vi "OpenVIs.vi"(8 "error in (no error)":errorcluster, 9 "Title Prefix In":string, 10 "VI Screenshots":T1, 11 "VI Path":path) -> (0 "error out":errorcluster, 2 "VI Screenshots out":T1)   [LabVIEW 2020, in "VIDiffUtilities.lvlib"]
uses:
  VIDiffUtilities.lvlib
  Screenshots/VIScreenshots.ctl
  Screenshots/ScreenshotInfo.ctl
  Screenshots/Screenshot Type.ctl
  FilePaths.ctl
  Screenshots/VIDiffScreenshots.lvlib
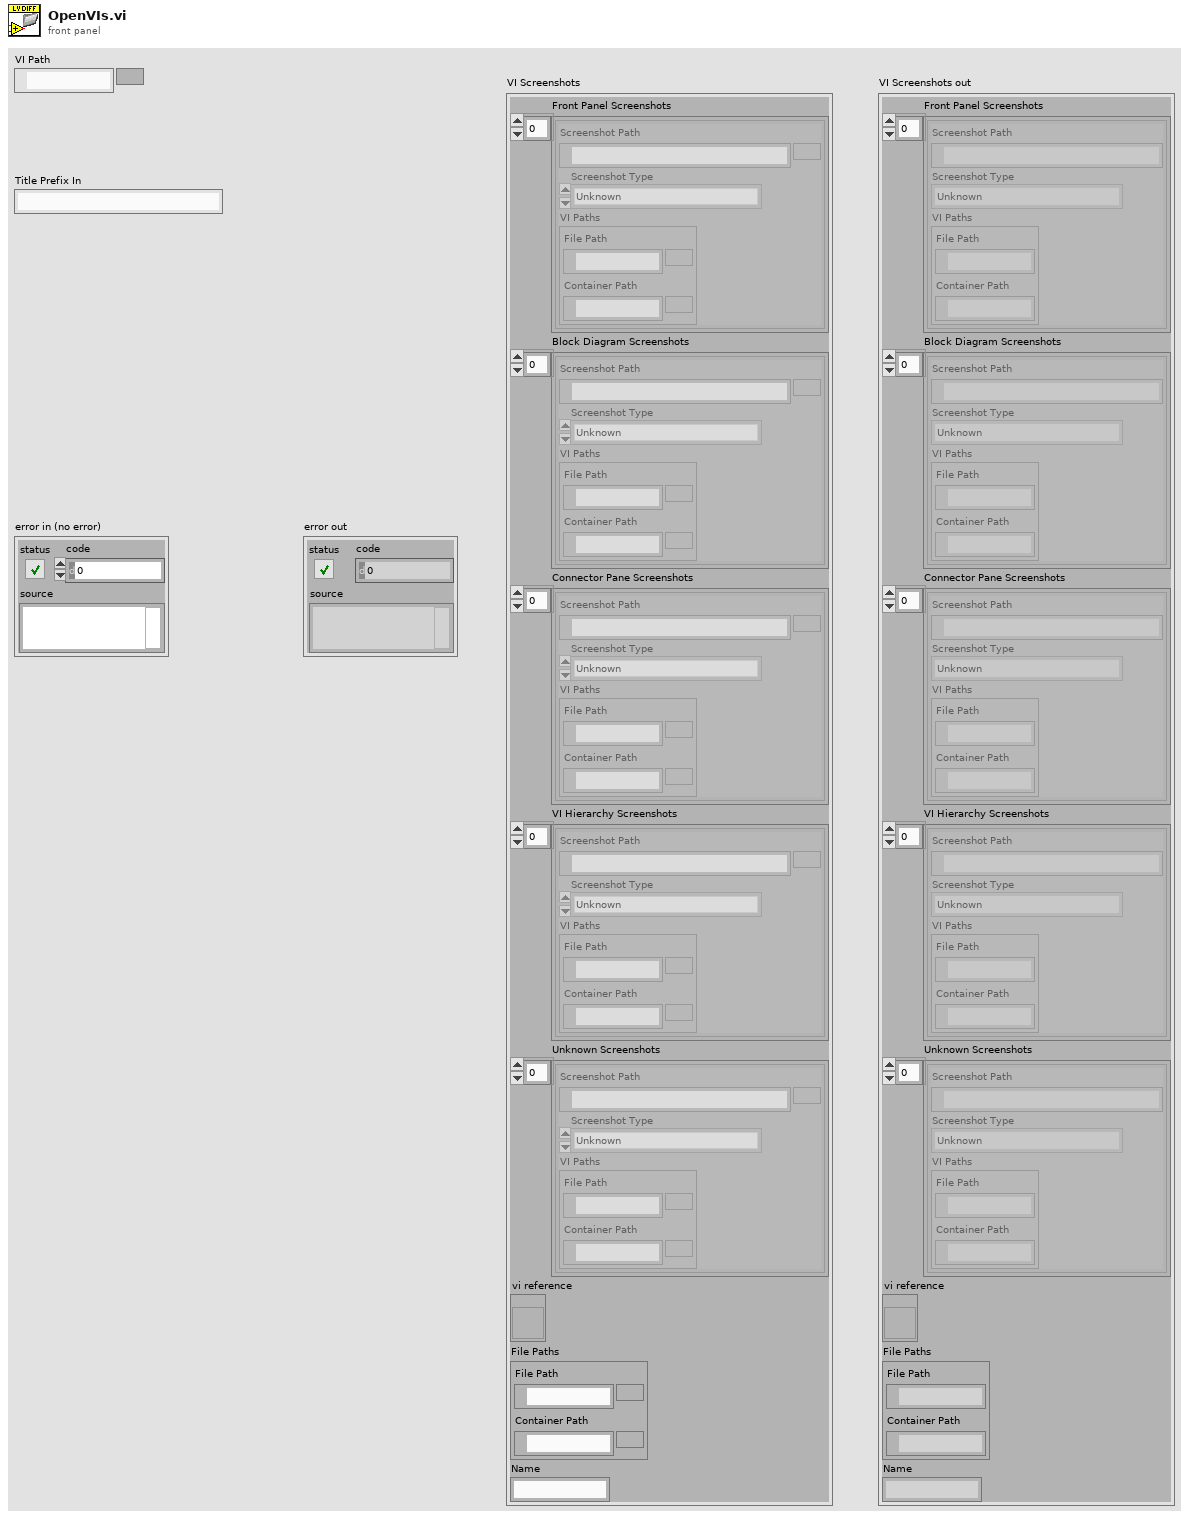
[diagram p1: front panel]
types:
  T1 = typedef "VIDiffScreenshots.lvlib/VIScreenshots.ctl" = cluster{"Front Panel Screenshots":T2[], "Block Diagram Screenshots":T2[], "Connector Pane Screenshots":T2[], "VI Hierarchy Screenshots":T2[], "Unknown Screenshots":T2[], "vi reference":refnum<vi>, "File Paths":cluster{"File Path":path, "Container Path":path}, "Name":string}
  T2 = typedef "VIDiffScreenshots.lvlib/ScreenshotInfo.ctl" = cluster{"Screenshot Path":path, "Screenshot Type":T3, "VI Paths":T4}
  T3 = typedef "VIDiffScreenshots.lvlib/Screenshot Type.ctl" = enum16{"Unknown", "Front Panel", "Connector Pane", "Block Diagram", "VI Hierarchy"}
  T4 = typedef "VIDiffUtilities.lvlib/FilePaths.ctl" = cluster{"File Path":path, "Container Path":path}
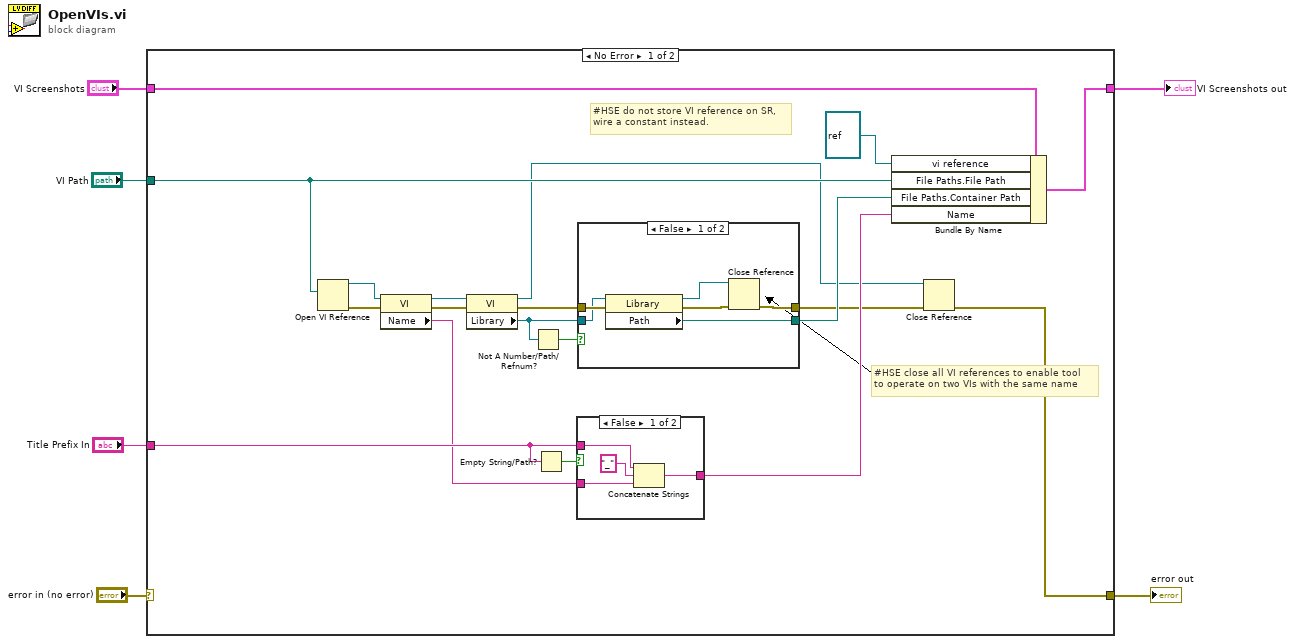
[diagram p0: block diagram]
diagram:
  n1 = case shown="No Error" "error in (no error)" {
    selector: "error in (no error)" -> [_ w39]
    tunnel: [w8 w39] -> w5
    tunnel: "VI Screenshots" -> [w22 w38]
    tunnel: [w20 w38] -> w3
    tunnel: "VI Path" -> [w19 _]
    tunnel: "Title Prefix In" -> [w13 _]
    frame No Error {
      # "#HSE do not store VI reference on SR,\nwire a constant instead."
      # "#HSE close all VI references to enable tool \nto operate on two VIs with the same name"
      n2 = Open VI Reference(vi path=w19) -> (vi reference=w18:refnum<vi>, error out=w17:errorcluster)  [unwired: 5 in]
      n3 = property class="VI"(reference=w18, error in=w17) -> (reference out=w15:refnum<vi>, error out=w16:errorcluster, "Name"=w12:string)
      n4 = property class="VI"(reference=w15, error in=w16) -> (reference out=w10:refnum<vi>, error out=w25:errorcluster, "Library"=w23:refnum<vi>)
      n5 = Not A Number/Path/Refnum?(number/path/refnum=w23) -> (NaN/Path/Refnum?=w24:bool)
      n6 = Empty String/Path?(string/path=w13) -> (empty?=w14:bool)
      n7 = case shown="False" w14 {
        tunnel: w12 -> [w29 w30]
        tunnel: [w28 w30] -> w11
        tunnel: w13 -> [w26 _]
        frame False {
          n8 = Concatenate Strings(w26, "_" ("string"), w29) -> (w28:string)
        }
        frame True {
        }
      }
      n9 = case shown="False" w24 {
        tunnel: [w36 _] -> w21
        tunnel: w25 -> [w35 w37]
        tunnel: [w31 w37] -> w9
        tunnel: w23 -> [w34 _]
        frame False {
          n10 = property class="Library"(reference=w34, error in=w35) -> (reference out=w33:refnum<vi>, error out=w32:errorcluster, "Path"=w36:path)
          n11 = Close Reference(reference=w33, error in (no error)=w32) -> (error out=w31:errorcluster)
        }
        frame True {
        }
      }
      n12 = Bundle By Name(cluster=w22, "vi reference"=refnum<vi> refnum, "File Paths.File Path"=w19, "File Paths.Container Path"=w21, "Name"=w11) -> (w20:T1)
      n13 = Close Reference(reference=w10, error in (no error)=w9) -> (error out=w8:errorcluster)
    }
    frame Error {
    }
  }
  "error out" <- w5
  "VI Screenshots out" <- w3
